vi "Analysis.Data Dump, Result Header to to 1D Str_V2a.vi"(7 "ValStr":variant, 10 "Result Summary":T1, 11 "Names":string[](array[string])) -> (3 "Data List out":string[](array[string]))   [LabVIEW 2024]
uses:
  Analysis.Result Summary_V2.ctl
  Time/Time.Format Selector.ctl
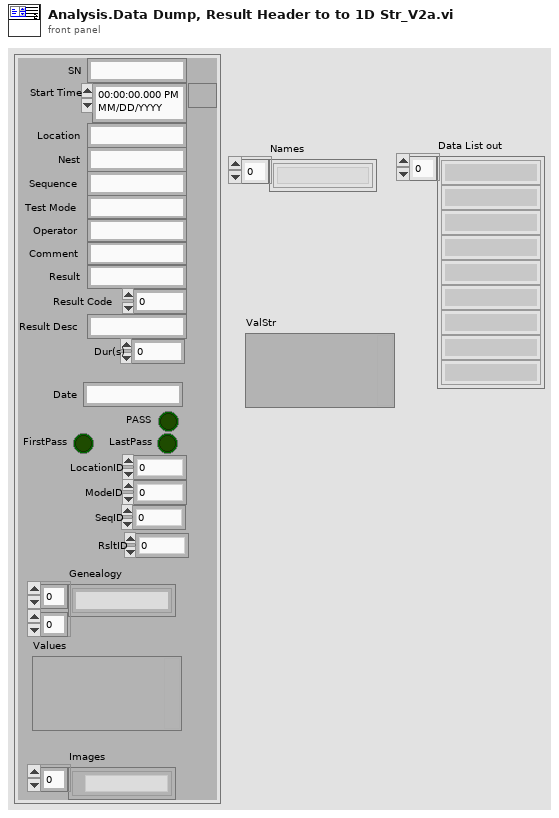
[diagram p1: front panel]
types:
  T1 = typedef "Analysis.Result Summary_V2.ctl" = cluster{"SN":string, "Start Time":timestamp, "Location":string, "Nest":string, "Sequence":string, "Operator":string, "Test Mode":string, "Comment":string, "Result":string, "Result Code":i32, "Result Desc":string, "Date":string, "Dur(s)":dbl, "PASS":bool, "FirstPass":bool, "LastPass":bool, "LocationID":i32, "ModeID":i32, "SeqID":i32, "RsltID":i32, "Genealogy":string[][], "Values":variant, "Images":path[]}
  T2 = typedef "Time.Format Selector.ctl" = enum16{"yyyy/mm/dd HH:MM:S.sss", "yyyy/mm/dd HH:MM:SS", "yyyy-MM-ddTHH:mm:ss[.mmm]", "YYYYMMDD_HHMMSS"}
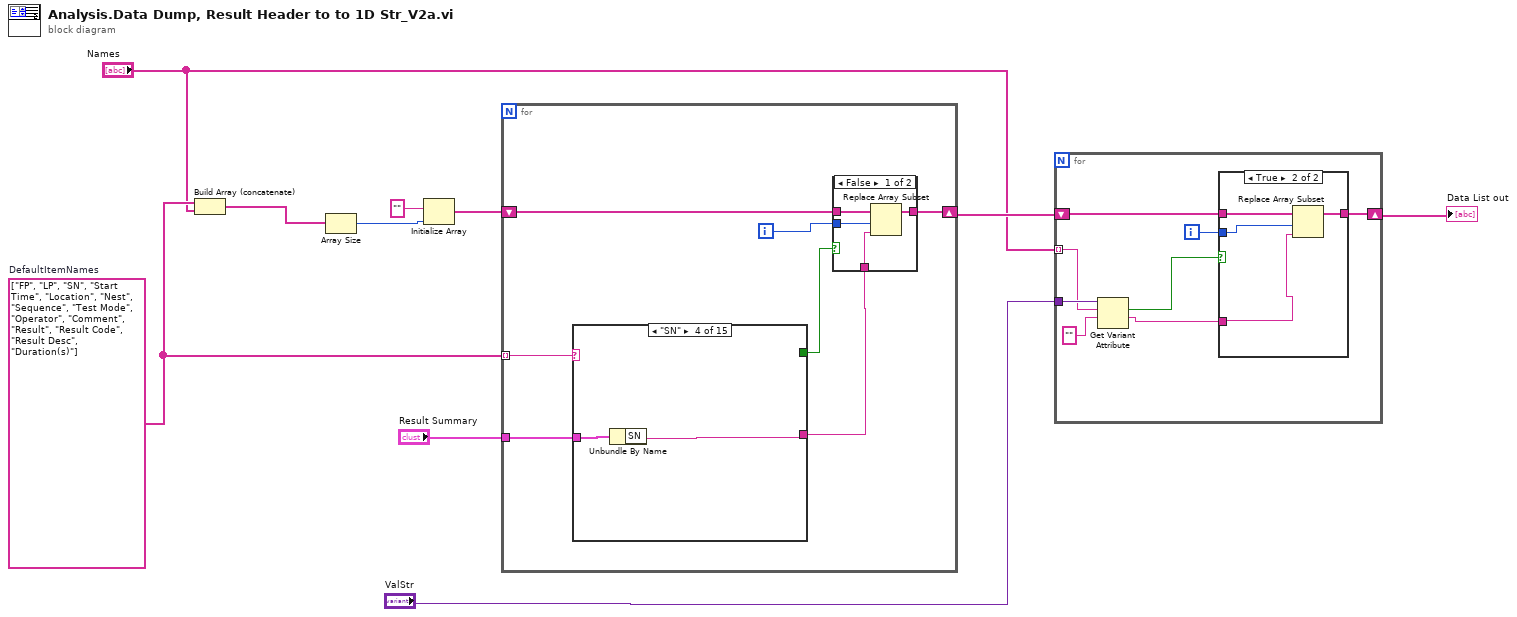
[diagram p0: block diagram]
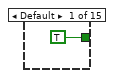
[diagram p4: hidden frame]
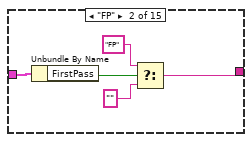
[diagram p5: hidden frame]
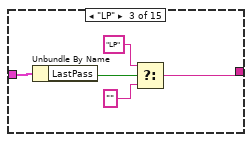
[diagram p6: hidden frame]
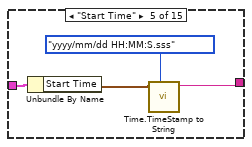
[diagram p7: hidden frame]
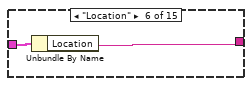
[diagram p8: hidden frame]
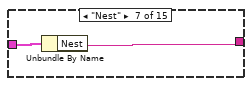
[diagram p9: hidden frame]
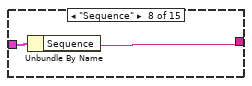
[diagram p10: hidden frame]
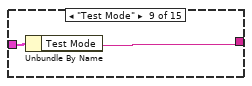
[diagram p11: hidden frame]
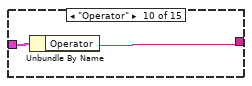
[diagram p12: hidden frame]
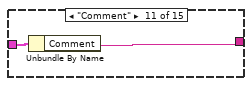
[diagram p13: hidden frame]
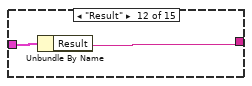
[diagram p14: hidden frame]
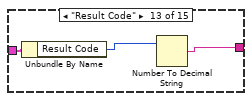
[diagram p15: hidden frame]
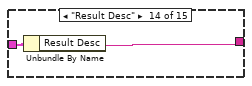
[diagram p16: hidden frame]
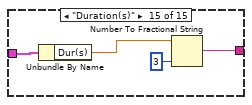
[diagram p17: hidden frame]
diagram:
  w5 = string[] ["FP", "LP", "SN", "Start Time", "Location", "Nest", "Sequence", "Test Mode", "Operator", "Comment", "Result", "Result Code", "Result Desc", "Duration(s)"]  # DefaultItemNames
  n1 = Build Array (concatenate)(w5, "Names") -> (w1:string[])
  n2 = Array Size(array=w1) -> (size(s)=w2:i32)
  n3 = Initialize Array("", w2) -> (w10:string[])
  n4 = for {
    shift-right: [w16] -> w8
    shift-left: w10 -> [w17]
    tunnel: "Result Summary" -> [w14]
    tunnel: w5 -> [w13] mode=indexing
    i -> [w12]
    n5 = case shown="\"SN\"" w13 {
      tunnel: [_ w26 w31 w34 w37 w40 w42 w44 w46 w48 w50 w52 w54 w57 w59] -> w15
      tunnel: w14 -> [_ w28 w33 w35 w39 w41 w43 w45 w47 w49 w51 w53 w56 w58 w62]
      tunnel: [TRUE _ _ _ _ _ _ _ _ _ _ _ _ _ _] -> w11
      frame Default {
      }
      frame "FP" {
        n6 = Unbundle By Name(w28) -> ("FirstPass"=w27:bool)
        n7 = Select(t="FP", s=w27, f="") -> (s? t:f=w26:string)
      }
      frame "LP" {
        n8 = Unbundle By Name(w33) -> ("LastPass"=w32:bool)
        n9 = Select(t="LP", s=w32, f="") -> (s? t:f=w31:string)
      }
      frame "SN" {
        n10 = Unbundle By Name(w35) -> ("SN"=w34:string)
      }
      frame "Start Time" {
        n11 = Unbundle By Name(w39) -> ("Start Time"=w38:timestamp)
        n12 = call "Time.TimeStamp to String.vi"("TimeFormat"=Time.Format_Selector."yyyy/mm/dd HH:MM:S.sss", "Time Stamp in"=w38) -> ("Time String Out"=w37:string)  [unwired: 9 in]
      }
      frame "Location" {
        n13 = Unbundle By Name(w41) -> ("Location"=w40:string)
      }
      frame "Nest" {
        n14 = Unbundle By Name(w43) -> ("Nest"=w42:string)
      }
      frame "Sequence" {
        n15 = Unbundle By Name(w45) -> ("Sequence"=w44:string)
      }
      frame "Test Mode" {
        n16 = Unbundle By Name(w47) -> ("Test Mode"=w46:string)
      }
      frame "Operator" {
        n17 = Unbundle By Name(w49) -> ("Operator"=w48:string)
      }
      frame "Comment" {
        n18 = Unbundle By Name(w51) -> ("Comment"=w50:string)
      }
      frame "Result" {
        n19 = Unbundle By Name(w53) -> ("Result"=w52:string)
      }
      frame "Result Code" {
        n20 = Unbundle By Name(w56) -> ("Result Code"=w55:i32)
        n21 = Number To Decimal String(number=w55) -> (decimal integer string=w54:string)  [unwired: 1 in]
      }
      frame "Result Desc" {
        n22 = Unbundle By Name(w58) -> ("Result Desc"=w57:string)
      }
      frame "Duration(s)" {
        n23 = Unbundle By Name(w62) -> ("Dur(s)"=w61:dbl)
        n24 = Number To Fractional String(number=w61, precision (6)=i16 3) -> (F-format string=w59:string)  [unwired: 2 in]
      }
    }
    n25 = case shown="False" w11 {
      tunnel: w17 -> [w21 w22]
      tunnel: [w20 w22] -> w16
      tunnel: w15 -> [w19 _]
      tunnel: w12 -> [w18 _]
      frame False {
        n26 = Replace Array Subset(array=w21, new element=w19, index=w18) -> (w20:string[])
      }
      frame True {
      }
    }
  }
  n27 = for {
    tunnel: "Names" -> [w66] mode=indexing
    shift-right: [w68] -> w7
    shift-left: w8 -> [w70]
    tunnel: "ValStr" -> [w67]
    i -> [w65]
    n28 = Get Variant Attribute(Variant=w67, name=w66, default value (empty Variant)="") -> (found=w69:bool, value=w64:string)  [unwired: 1 in, 2 out]
    n29 = case shown="True" w69 {
      tunnel: w70 -> [w71 w75]
      tunnel: [w71 w74] -> w68
      tunnel: w65 -> [_ w73]
      tunnel: w64 -> [_ w72]
      frame False {
      }
      frame True {
        n30 = Replace Array Subset(array=w75, new element=w72, index=w73) -> (w74:string[])
      }
    }
  }
  "Data List out" <- w7
